vi "InsertNodes.vi"(6 "InsertSearch":T1={"GraphSearch"=refnum, "InsertIfEmpty"=TRUE}, 8 "error in (no error)":errorcluster, 9 "position":T2=enum."Search", 10 "ToInsert":refnum<data-value>, 11 "Graph in":refnum<class "Graph.lvclass">) -> (0 "error out":errorcluster, 1 "ignored":bool, 3 "Graph out":refnum<class "Graph.lvclass">)   [LabVIEW 2009, in "Graph.lvclass"]
uses:
  Graph.lvclass
  GraphNode/GraphNode.lvclass
  GraphSearch/GraphSearch.lvclass
  position.ctl
  InsertSearch.ctl
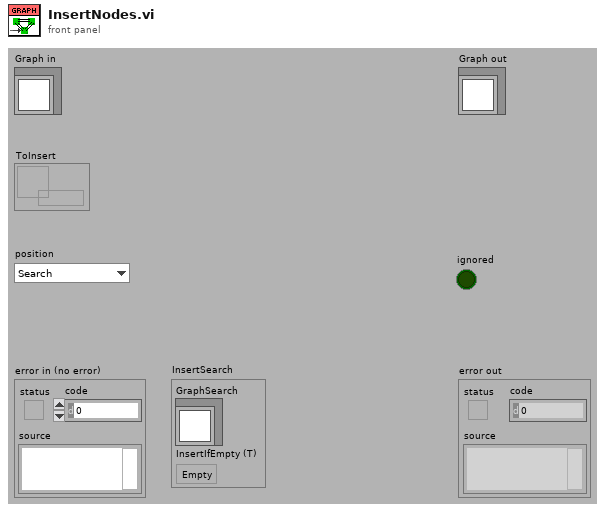
[diagram p1: front panel]
types:
  T1 = typedef "Graph.lvclass/InsertSearch.ctl" = cluster{"GraphSearch":refnum<class "GraphSearch.lvclass">, "InsertIfEmpty":bool}
  T2 = typedef "Graph.lvclass/position.ctl" = enum16{"Link To All", "Search"}
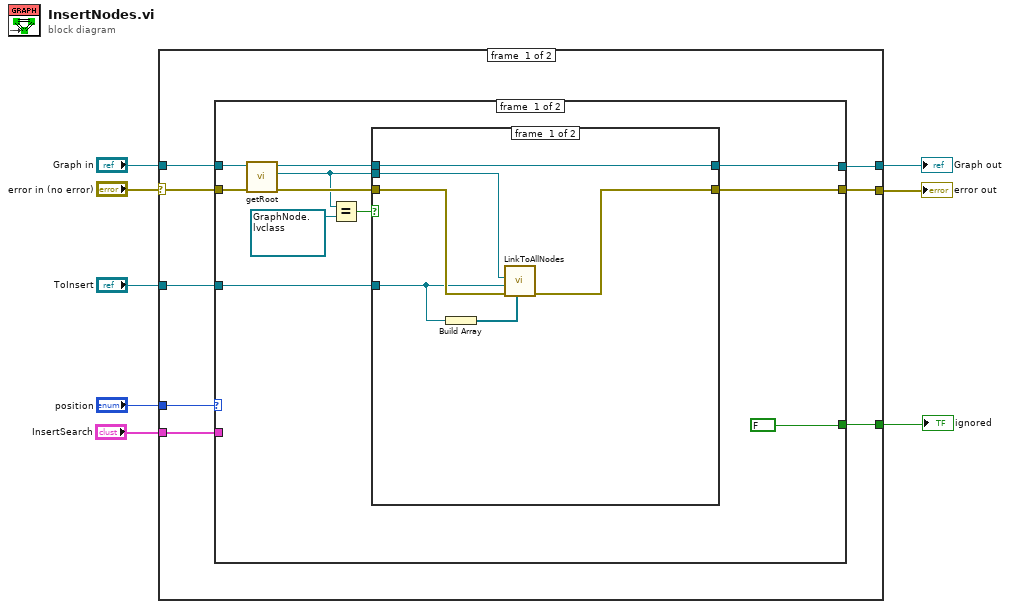
[diagram p0: block diagram]
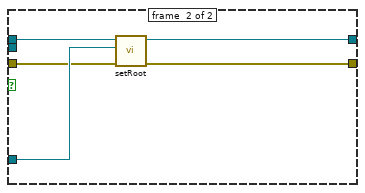
[diagram p2: hidden frame]
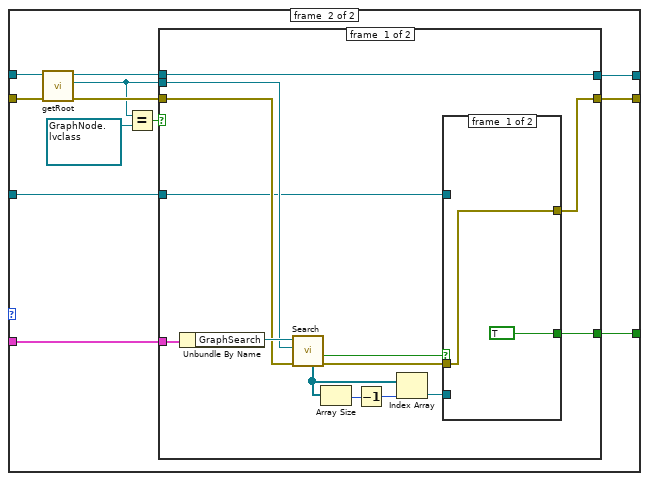
[diagram p3: hidden frame]
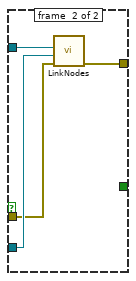
[diagram p4: hidden frame]
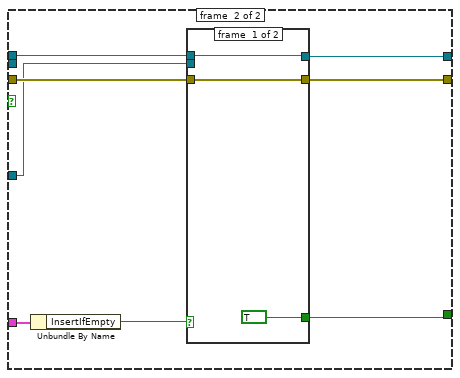
[diagram p5: hidden frame]
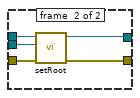
[diagram p6: hidden frame]
diagram:
  n1 = case shown="No Error" "error in (no error)" {
    selector: "error in (no error)" -> [w12 w88]
    tunnel: [w9 w88] -> w7
    tunnel: [w10 w87] -> w5
    tunnel: "Graph in" -> [w13 w87]
    tunnel: "ToInsert" -> [w11 _]
    tunnel: "InsertSearch" -> [w15 _]
    tunnel: "position" -> [w16 _]
    tunnel: [w14 _] -> w1
    frame #0 {
      n2 = case shown="\"Search\", Default" w16 {
        tunnel: w13 -> [w26 w50]
        tunnel: w12 -> [w25 w49]
        tunnel: w15 -> [_ w45]
        tunnel: w11 -> [w20 w43]
        tunnel: [w19 w41] -> w10
        tunnel: [w21 w40] -> w9
        tunnel: [FALSE w39] -> w14
        frame #0 {
          n3 = call "getRoot.vi"("error in (no error)"=w25, "Graph in"=w26) -> ("error out"=w22:errorcluster, "Root"=w17:refnum<data-value>, "Graph out"=w24:refnum<class "Graph.lvclass">)  [unwired: 7 in]
          n4 = Equal?(x=w17, y=refnum<data-value> refnum) -> (x = y?=w23:bool)
          n5 = case shown="False" w23 {
            tunnel: w24 -> [w33 w38]
            tunnel: w22 -> [w32 w36]
            tunnel: [w28 w34] -> w21
            tunnel: w20 -> [w30 w37]
            tunnel: [w33 w35] -> w19
            tunnel: w17 -> [w31 _]
            frame #0 {
              n6 = Build Array(w30) -> (w29:refnum<data-value>[])
              n7 = call "LinkToAllNodes.vi"("NodeList in"=w29, "error in (no error)"=w32, "GraphNode2 in"=w30, "GraphNode1 in"=w31) -> ("error out"=w28:errorcluster)  [unwired: 4 in, 3 out]
            }
            frame #1 {
              n8 = call "setRoot.vi"("error in (no error)"=w36, "Root"=w37, "Graph in"=w38) -> ("error out"=w34:errorcluster, "Graph out"=w35:refnum<class "Graph.lvclass">)  [unwired: 7 in]
            }
          }
        }
        frame #1 {
          n9 = call "getRoot.vi"("error in (no error)"=w49, "Graph in"=w50) -> ("error out"=w46:errorcluster, "Root"=w44:refnum<data-value>, "Graph out"=w47:refnum<class "Graph.lvclass">)  [unwired: 7 in]
          n10 = Equal?(x=w44, y=refnum<data-value> refnum) -> (x = y?=w48:bool)
          n11 = case shown="False" w48 {
            tunnel: w47 -> [w55 w77]
            tunnel: w46 -> [w61 w76]
            tunnel: w45 -> [w64 w78]
            tunnel: w44 -> [w62 _]
            tunnel: w43 -> [w56 w75]
            tunnel: [w55 w73] -> w41
            tunnel: [w54 w72] -> w40
            tunnel: [w53 w71] -> w39
            frame #0 {
              n12 = Unbundle By Name(w64) -> ("GraphSearch"=w63:refnum<class "GraphSearch.lvclass">)
              n13 = call "Search.vi"("error in (no error)"=w61, "FirstNode in"=w62, "GraphSearch in"=w63) -> ("error out"=w58:errorcluster, "found"=w59:bool, "Path"=w60:refnum<data-value>[])  [unwired: 5 in, 1 out]
              n14 = Array Size(array=w60) -> (size(s)=w51:i32)
              n15 = Decrement(x=w51) -> (x-1=w52:i32)
              n16 = Index Array(array=w60, index=w52) -> (element=w57:refnum<data-value>)
              n17 = case shown="True" w59 {
                tunnel: w58 -> [w66 w68]
                tunnel: w57 -> [_ w69]
                tunnel: w56 -> [_ w70]
                tunnel: [w66 w67] -> w54
                tunnel: [TRUE _] -> w53
                frame #0 {
                }
                frame #1 {
                  n18 = call "LinkNodes.vi"("error in (no error)"=w68, "GraphNode2 in"=w69, "GraphNode1 in"=w70) -> ("error out"=w67:errorcluster)  [unwired: 6 in, 2 out]
                }
              }
            }
            frame #1 {
              n19 = Unbundle By Name(w78) -> ("InsertIfEmpty"=w74:bool)
              n20 = case shown="True" w74 {
                tunnel: w77 -> [w81 w86]
                tunnel: w76 -> [w80 w85]
                tunnel: w75 -> [_ w84]
                tunnel: [w81 w83] -> w73
                tunnel: [w80 w82] -> w72
                tunnel: [TRUE _] -> w71
                frame #0 {
                }
                frame #1 {
                  n21 = call "setRoot.vi"("error in (no error)"=w85, "Root"=w84, "Graph in"=w86) -> ("error out"=w82:errorcluster, "Graph out"=w83:refnum<class "Graph.lvclass">)  [unwired: 7 in]
                }
              }
            }
          }
        }
      }
    }
    frame #1 {
    }
  }
  "error out" <- w7
  "Graph out" <- w5
  "ignored" <- w1
